vi "pane color.vi"() -> ()   [LabVIEW 2016]
panel:
  out "Round Color Box 2":u32 format="%x"
  in  "Round Color Box":u32(colorbox)
  out "number":i32
  in  "String 3":string
  out "concatenated string":string
  in  "String 2":string
  in  "String":string
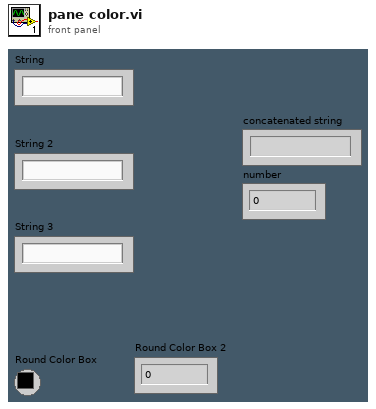
[diagram p1: front panel]
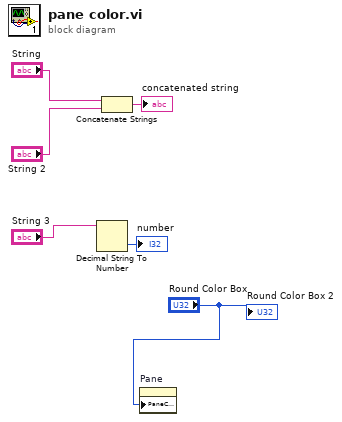
[diagram p0: block diagram]
diagram:
  n1 = Decimal String To Number(string="String 3") -> (number=→"number":i32)  [unwired: 2 in, 1 out]
  n2 = Concatenate Strings("String", "String 2") -> (→"concatenated string":string)
  n3 = property on="Pane" class="Pane"("PaneColor"="Round Color Box") -> ()  [unwired: 2 in, 2 out]
  "Round Color Box 2" <- "Round Color Box"
